vi "Hardware - Trigger Timestamp.vi"(8 "error in (no error)":errorcluster) -> (0 "error out":errorcluster, 3 "Timer Value (ms)":dbl caption="Time Value (ms)" format="%#.6g")   [LabVIEW 2010, in "Core SubVIs.lvlib"]
uses:
  Core SubVIs.lvlib
  Controls/TYPE - Count Time Method.ctl
  <vilib>/DAQmx/write.llb/DAQmx Write (Digital Bool 1Line 1Point).vi
  <vilib>/Waveform/DWDTOps.llb/Digital Pattern Generator (Toggle).vi
  <vilib>/daqmx/miscellaneous.llb/DAQmx Fill In Error Info.vi
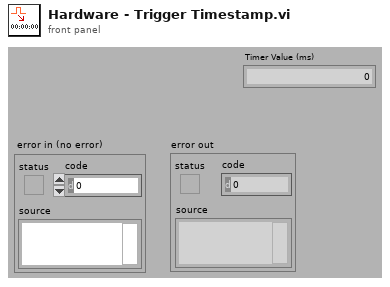
[diagram p1: front panel]
types:
  T1 = typedef "Core SubVIs.lvlib/TYPE - Count Time Method.ctl" = enum16{"Start Timer Task", "Read Timer", "Reset Timer", "Clear Timer Task"}
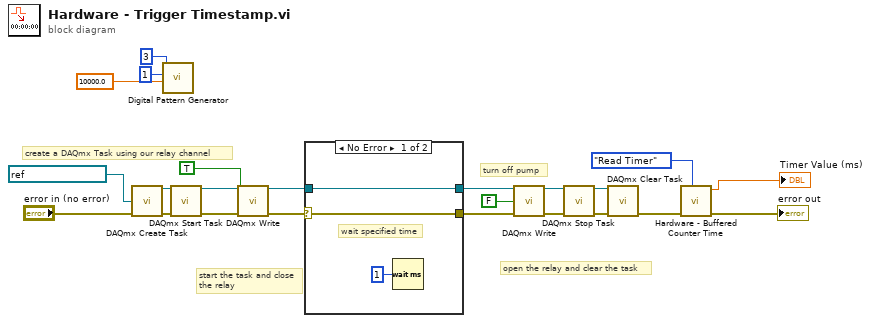
[diagram p0: block diagram]
diagram:
  # "open the relay and clear the task"
  # "start the task and close\nthe relay"
  # "create a DAQmx Task using our relay channel"
  # "turn off pump"
  n1 = call <vilib>:"DAQmx Create Task.vi"("global virtual channels"=refnum<k21> "EVENT_1_OUT", "error in"="error in (no error)") -> ("task out"=w22:refnum<k21>, "error out"=w21:errorcluster)  [unwired: 3 in, 9 out]
  n2 = call-poly <vilib>:"Digital Pattern Generator.vi"("sample rate"=10000.0, "number of signals"=u32 1, "number of samples"=u32 3) -> ()  [unwired: 3 in, 6 out]
  n3 = call <vilib>:"DAQmx Start Task.vi"("task/channels in"=w22, "error in"=w21) -> ("task out"=w19:refnum<k21>, "error out"=w20:errorcluster)  [unwired: 12 out]
  n4 = call-poly <vilib>:"DAQmx Write.vi"("task/channels in"=w19, "data"=TRUE, "error in"=w20) -> ("task out"=w13:refnum<k21>, "error out"=w12:errorcluster)  [unwired: 1 in, 10 out]
  n5 = case shown="No Error" w12 {
    selector: w12 -> [w26 w27]
    tunnel: w13 -> [w25 w28]
    tunnel: [w26 w27] -> w11
    tunnel: [w25 w28] -> w10
    frame No Error {
      # "wait specified time"
      n6 = Wait (ms)(milliseconds to wait=u32 1) -> ()  [unwired: 1 out]
    }
    frame Error {
    }
  }
  n7 = call-poly <vilib>:"DAQmx Write.vi"("task/channels in"=w10, "data"=FALSE, "error in"=w11) -> ("task out"=w17:refnum<k21>, "error out"=w16:errorcluster)  [unwired: 1 in, 10 out]
  n8 = call <vilib>:"DAQmx Stop Task.vi"("task/channels in"=w17, "error in"=w16) -> ("task out"=w15:refnum<k21>, "error out"=w14:errorcluster)  [unwired: 12 out]
  n9 = call <vilib>:"DAQmx Clear Task.vi"("task in"=w15, "error in"=w14) -> ("error out"=w8:errorcluster)  [unwired: 13 out]
  n10 = call "Hardware - Buffered Counter Time.vi"("Counter Time Function (Read Timer)"=TYPE_-_Count_Time_Method."Read Timer", "error in (no error)"=w8) -> ("error out"=→"error out":errorcluster, "Timer Value (ms)"=→"Timer Value (ms)":dbl)  [unwired: 1 in, 7 out]
